vi "sBeam loggen.vi"(8 "error in (no error)":errorcluster caption="Fehler (Eingang, kein Fehler)") -> (0 "error out":errorcluster caption="Fehler (Ausgang)")   [LabVIEW 2020, in "FT-IR.lvlib"]
uses:
  FT-IR.lvlib
  FGV FT-IR Diagnose Aktionen.ctl
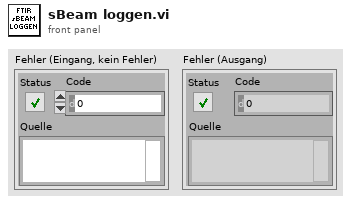
[diagram p1: front panel]
types:
  T1 = typedef "FT-IR.lvlib/FGV FT-IR Diagnose Aktionen.ctl" = enum16{"Lesen", "Diagnose Schreiben", "Min Schreiben", "Max Schreiben"}
  T2 = enum16{"open", "replace", "create", "open or create", "replace or create", "replace or create with confirmation"}
  T3 = typedef "FT-IR.lvlib/TOOLweb Interface.lvlib/Typdefinitionen.lvlib/TOOLweb Diagnose.ctl" = cluster{"(14) temperature":sgl, "(15) pressure":sgl, "(16) oxygen":sgl, "(50) diag-igramdc":sgl, "(51) diag-igrampp":sgl, "(52) diag-phaseAngle":sgl, "(53) diag-laserpp":sgl, "(54) diag-laserdc":sgl, "(55) diag-badscan":sgl, "(56) diag-centerburst":sgl, "(57) diag-linearizerCheck":sgl, "(58) diag-SNR":sgl, "(59) diag-sBeamIntensity":sgl}
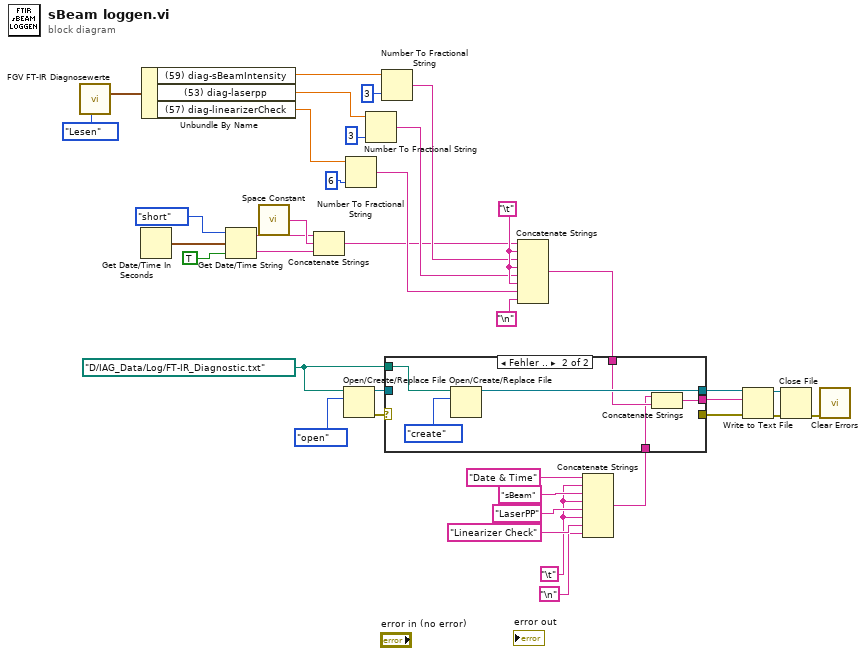
[diagram p0: block diagram]
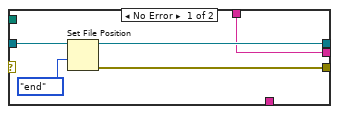
[diagram p2: hidden frame]
diagram:
  w2 = "\t"
  w17 = "\t"
  w12 = path "D:/IAG_Data/Log/FT-IR_Diagnostic.txt" ("Dateipfad (Dialog verwenden)")
  n1 = call "FGV FT-IR Diagnosewerte.vi"("Aktionen"=FGV_FT-IR_Diagnose_Aktionen."Lesen") -> ("Diagnose"=w33:T3)  [unwired: 5 in, 5 out]
  n2 = Get Date/Time In Seconds() -> (seconds since 1Jan1904=w27:timestamp)
  n3 = Unbundle By Name(w33) -> ("(59) diag-sBeamIntensity"=w26:sgl, "(53) diag-laserpp"=w23:sgl, "(57) diag-linearizerCheck"=w18:sgl)
  n4 = Get Date/Time String(date format (0)=enum16{"short", "long", "abbreviated"}."short" ("Datumsformat (0)"), seconds (now)=w27, want seconds? (F)=TRUE ("Angabe von Sekunden? (F)")) -> (date string=w30:string, time string=w32:string)
  n5 = call <vilib>:"Space Constant.vi"() -> ("String"=w31:string)
  n6 = Concatenate Strings(w30, w31, w32) -> (w13:string)
  n7 = Open/Create/Replace File(file path (use dialog)=w12, operation (0:open)=T2."open" ("Operation (0:Öffnen)")) -> (refnum out=w21:refnum<file>, error out=w22:errorcluster)  [unwired: 4 in, 1 out]
  n8 = Number To Fractional String(number=w18, precision (6)=i16 6 ("Breite (-)")) -> (F-format string=w15:string)  [unwired: 2 in]
  n9 = Number To Fractional String(number=w23, precision (6)=i16 3 ("Breite (-)")) -> (F-format string=w16:string)  [unwired: 2 in]
  n10 = Number To Fractional String(number=w26, precision (6)=i16 3 ("Breite (-)")) -> (F-format string=w14:string)  [unwired: 2 in]
  n11 = Concatenate Strings(w13, w17, w14, w17, w16, w17, w15, "\n") -> (w5:string)
  n12 = Concatenate Strings("Date & Time" ("String"), w2, "sBeam" ("String"), w2, "LaserPP" ("String"), w2, "Linearizer Check" ("String"), "\n") -> (w4:string)
  n13 = case shown="Fehler .." w22 {
    tunnel: w21 -> [w43 _]
    tunnel: [w42 w49] -> w20
    tunnel: w12 -> [_ w48]
    tunnel: [w41 _] -> w11
    tunnel: [w39 w46] -> w6
    tunnel: w5 -> [w39 w45]
    tunnel: w4 -> [_ w44]
    frame No Error {
      n14 = Set File Position(refnum=w43, from (0:start)=enum16{"start", "end", "current"}."end" ("Von (0:Start)")) -> (refnum out=w42:refnum<file>, error out=w41:errorcluster)  [unwired: 2 in]
    }
    frame Error {
      n15 = Open/Create/Replace File(file path (use dialog)=w48, operation (0:open)=T2."create" ("Operation (0:Öffnen)")) -> (refnum out=w49:refnum<file>)  [unwired: 4 in, 2 out]
      n16 = Concatenate Strings(w44, w45) -> (w46:string)
    }
  }
  n17 = Write to Text File(file (use dialog)=w20, text=w6, error in=w11) -> (refnum out=w37:refnum<file>, error out=w38:errorcluster)  [unwired: 1 in, 1 out]
  n18 = Close File(refnum=w37, error in=w38) -> (error out=w36:errorcluster)  [unwired: 1 out]
  n19 = call <vilib>:"Clear Errors.vi"("error in (no error)"=w36) -> ()  [unwired: 5 in, 2 out]
